vi "SVT THD and Harmonic Components (Frequency) (1 Ch).vi"(0 "complex spectrum":T9={"complex spectrum response"={"f0"=0.0, "df"=1.0, "complex spectrum"=[]}, "spectrum info"={"channel name"="", "description"="", "x-axis units"=0, "spectral info"={"spectrum type"=enum."Power [Magnitude^2]", "linear/dB"=enum."linear", "window"=0, "window size"=0, "FFT size"=0}, "engineering units"=0, "custom label"="", "dB reference [EU]"=0.0, "peak units"=enum."rms", "weighting filter"=0, "spectral density?"=FALSE, "unit label"="", "spectrum skewed?"=FALSE, "complimentary spectrum units"=enum."none"}} {"spectrum info"."x-axis units" items=["Time (s)"=0, "Frequency-CB (Hz)"=1, "Frequency-CPB (Hz)"=1248, "Frequency-Arbitrary (Hz)"=2357, "Quefrency (s)"=2, "Revolutions (rev)"=3, "Order"=4, "Speed (RPM)"=11, "Speed (rad/s)"=21, "Index"=65535]; "spectrum info"."weighting filter" items=["Linear", "A-weighting", "B-weighting", "C-weighting", "ITU-R 468-4", "Dolby", "CCITT", "C-message", "Wb", "Wc", "Wd", "We", "Wf", "Wh", "Wj", "Wk", "Wm", "AES17 20 kHz lowpass", "AES17 40 kHz lowpass", "AES17 20 kHz highpass", "AES17 40 kHz highpass"]; "spectrum info"."dB reference [EU]" format="%.2f"; "spectrum info"."engineering units" items=["custom..."=0, "V"=1, "A"=21, "C"=30, "pC"=31, "s"=32, "-"=29, "Pa"=2, "N"=20, "g"=3, "m/s^2"=4, "m/s"=5, "m"=6, "mm/s"=12, "mm"=13, "micron/s"=14, "micron"=15, "in/s^2"=7, "in/s"=8, "in"=9, "mil/s"=10, "mil"=11, "rad/s^2"=16, "rad/s"=17, "rad"=18, "deg/s^2"=26, "deg/s"=27, "deg"=28, "RPM"=22, "cycle/s^2"=23, "Hz"=24, "cycle"=25, "strain"=19]; "spectrum info"."spectral info"."window" items=["None "=0, "Hanning"=1, "Hamming"=2, "Blackman-Harris"=3, "Exact Blackman"=4, "Blackman"=5, "Flat Top"=6, "4 Term B-Harris "=7, "7 Term B-Harris"=8, "Low Sidelobe"=9, "Force - Exponential"=10, "Gaussian"=62]; "complex spectrum response"."complex spectrum" format="%.2f"; "complex spectrum response"."df" format="%.2f"; "complex spectrum response"."f0" format="%.2f"}, 2 "maximum harmonic":i32=-1, 3 "harmonics to visualize":i32[](array[numeric])=[-1], 5 "error in (no error)":errorcluster, 6 "desired units":T2, 9 "expected fundamental frequency [Hz]":dbl=-1.0 format="%.2f") -> (10 "actual maximum harmonic":i32=5, 11 "detected fundamental\nfrequency [Hz]":dbl format="%.2f", 12 "unit labels":T1, 13 "detected fundamental\namplitude":dbl format="%.2f", 14 "complex spectrum":T9={"complex spectrum response"={"f0"=0.0, "df"=1.0, "complex spectrum"=[]}, "spectrum info"={"channel name"="", "description"="", "x-axis units"=0, "spectral info"={"spectrum type"=enum."Power [Magnitude^2]", "linear/dB"=enum."linear", "window"=0, "window size"=0, "FFT size"=0}, "engineering units"=0, "custom label"="", "dB reference [EU]"=0.0, "peak units"=enum."rms", "weighting filter"=0, "spectral density?"=FALSE, "unit label"="", "spectrum skewed?"=FALSE, "complimentary spectrum units"=enum."none"}} {"spectrum info"."x-axis units" items=["Time (s)"=0, "Frequency-CB (Hz)"=1, "Frequency-CPB (Hz)"=1248, "Frequency-Arbitrary (Hz)"=2357, "Quefrency (s)"=2, "Revolutions (rev)"=3, "Order"=4, "Speed (RPM)"=11, "Speed (rad/s)"=21, "Index"=65535]; "spectrum info"."weighting filter" items=["Linear", "A-weighting", "B-weighting", "C-weighting", "ITU-R 468-4", "Dolby", "CCITT", "C-message", "Wb", "Wc", "Wd", "We", "Wf", "Wh", "Wj", "Wk", "Wm", "AES17 20 kHz lowpass", "AES17 40 kHz lowpass", "AES17 20 kHz highpass", "AES17 40 kHz highpass"]; "spectrum info"."dB reference [EU]" format="%.2f"; "spectrum info"."engineering units" items=["custom..."=0, "V"=1, "A"=21, "C"=30, "pC"=31, "s"=32, "-"=29, "Pa"=2, "N"=20, "g"=3, "m/s^2"=4, "m/s"=5, "m"=6, "mm/s"=12, "mm"=13, "micron/s"=14, "micron"=15, "in/s^2"=7, "in/s"=8, "in"=9, "mil/s"=10, "mil"=11, "rad/s^2"=16, "rad/s"=17, "rad"=18, "deg/s^2"=26, "deg/s"=27, "deg"=28, "RPM"=22, "cycle/s^2"=23, "Hz"=24, "cycle"=25, "strain"=19]; "spectrum info"."spectral info"."window" items=["None "=0, "Hanning"=1, "Hamming"=2, "Blackman-Harris"=3, "Exact Blackman"=4, "Blackman"=5, "Flat Top"=6, "4 Term B-Harris "=7, "7 Term B-Harris"=8, "Low Sidelobe"=9, "Force - Exponential"=10, "Gaussian"=62]; "complex spectrum response"."complex spectrum" format="%.2f"; "complex spectrum response"."df" format="%.2f"; "complex spectrum response"."f0" format="%.2f"}, 16 "THD":dbl format="%.2f", 17 "harmonic components":cluster{"frequency [Hz]":dbl, "amplitude":dbl}[](array[cluster]) {"amplitude" format="%.2f"; "frequency [Hz]" format="%.2f"}, 19 "error out":errorcluster)   [LabVIEW 2017, in "SoundVib_Distortion.lvlib"]
doc: "Performs a total harmonic distortion analysis, including measuring the fundamental tone and harmonics, and returns the detected fundamental frequency, detected fundamental amplitude, harmonic components, and total harmonic distortion (THD). Wire data to the <B>scaled signal [EU]</B> input to determine the polymorphic instance to use or manually select the instance.\n\nThe following formula calculates THD:\n\nTHD = H / F\n\nwhere H is the harmonic RMS level and F is the fundamental tone RMS level."
uses:
  <vilib>/addons/Sound and Vibration/svt_Distortion/SoundVib_Distortion.lvlib
  <vilib>/addons/_NISVFA/_Shared subVIs/Controls/svc_Spectrum Info.ctl
  <vilib>/addons/_NISVFA/_Shared subVIs/Controls/svc_X-Axis Units.ctl
  <vilib>/addons/_NISVFA/_Shared subVIs/Controls/svc_Spectrum Type.ctl
  <vilib>/addons/_NISVFA/_Shared subVIs/Controls/svc_Engineering Units Text Ring.ctl
  <vilib>/addons/_NISVFA/_Shared subVIs/Controls/svc_Weighting Filter Text Ring.ctl
  <vilib>/addons/_NISVFA/_Shared subVIs/Controls/svc_Complimentary Spectrum Units.ctl
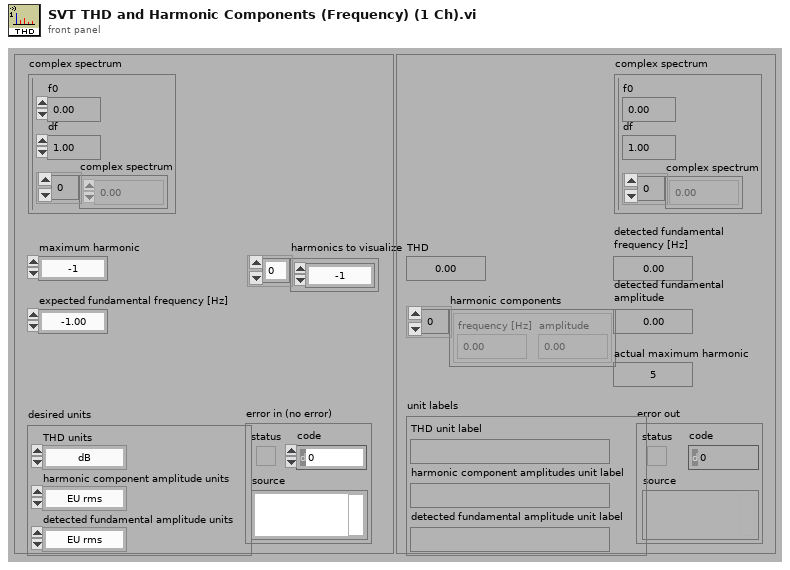
[diagram p1: front panel]
types:
  T1 = cluster{"THD unit label":string, "harmonic component amplitudes unit label":string, "detected fundamental amplitude unit label":string}
  T2 = cluster{"THD units":enum16{"dB", "linear ratio", "%"}, "harmonic component amplitude units":enum16{"EU rms", "EU peak", "EU peak-peak", "dB ref fund"}, "detected fundamental amplitude units":enum16{"EU rms", "EU peak", "EU peak-peak"}}
  T3 = typedef "svc_Spectrum Info.ctl" = cluster{"channel name":string, "description":string, "x-axis units":T4, "spectral info":cluster{"spectrum type":T5, "linear/dB":enum16{"linear", "dB"}, "window":u16, "window size":i32, "FFT size":i32}, "engineering units":T6, "custom label":string, "dB reference [EU]":dbl, "peak units":enum16{"rms", "peak", "peak-peak"}, "weighting filter":T7, "spectral density?":bool, "unit label":string, "spectrum skewed?":bool, "complimentary spectrum units":T8}
  T4 = typedef "svc_X-Axis Units.ctl" = u16
  T5 = typedef "svc_Spectrum Type.ctl" = enum16{"FFT Spectrum [complex]", "Amplitude [Magnitude]", "Power [Magnitude^2]", "Cross Spectrum [complex]", "Frequency Response [Complex]"}
  T6 = typedef "svc_Engineering Units Text Ring.ctl" = u16
  T7 = typedef "svc_Weighting Filter Text Ring.ctl" = u16
  T8 = typedef "svc_Complimentary Spectrum Units.ctl" = enum16{"none", "radians", "degrees", "cycles", "imaginary"}
  T9 = cluster{"complex spectrum response":cluster{"f0":dbl, "df":dbl, "complex spectrum":cdb[]}, "spectrum info":T3}
  T10 = cluster{"unit label":string, "unit label":string, "unit label":string}
  T11 = enum16{"EU rms", "EU peak", "EU peak-peak", "dB ref fund"}
  T12 = cluster{"SINAD [ratio]":dbl, "THD+N [ratio]":dbl, "THD":dbl}
  T13 = cluster{"detected frequency [Hz]":dbl, "detected amplitude":dbl}[]
  T14 = cluster{"frequency [Hz]":dbl, "converted harmonic amplitude":dbl}
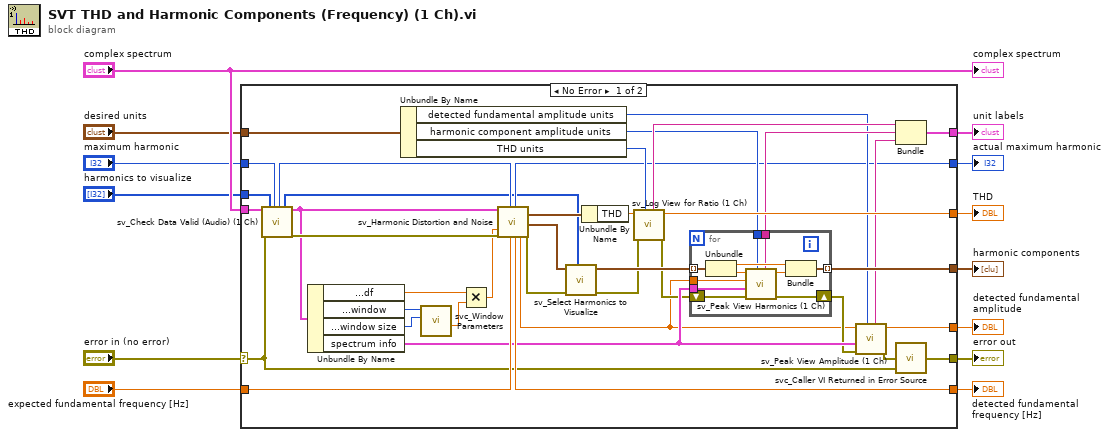
[diagram p0: block diagram]
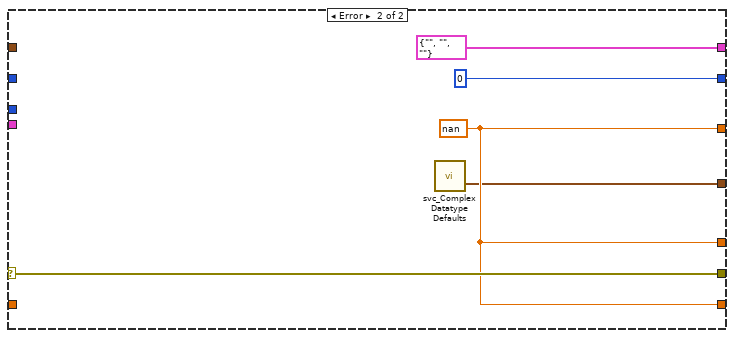
[diagram p2: hidden frame]
diagram:
  n1 = case shown="No Error" "error in (no error)" {
    selector: "error in (no error)" -> [w20 w68]
    tunnel: "complex spectrum" -> [w32 _]
    tunnel: "expected fundamental frequency [Hz]" -> [w52 _]
    tunnel: [w49 w68] -> w12
    tunnel: [w45 w67] -> w11
    tunnel: [w39 w64] -> w6
    tunnel: [w51 w67] -> w9
    tunnel: [w48 w67] -> w7
    tunnel: "maximum harmonic" -> [w33 _]
    tunnel: "harmonics to visualize" -> [w34 _]
    tunnel: "desired units" -> [w47 _]
    tunnel: [w36 T10 {"unit label"="", "unit label"="", "unit label"=""}] -> w2
    tunnel: [w35 0 ("actual maximum harmonic")] -> w1
    frame No Error {
      n2 = call <vilib>:"sv_Check Data Valid (Audio) (1 Ch).vi"("complex spectrum"=w32, "error in (no error)"=w20, "harmonics to visualize"=w34, "maximum harmonic"=w33) -> ("dup maximum harmonic"=w31:i32, "dup harmonics to visualize"=w27:i32[], "complex spectrum"=w28:T9, "error out"=w30:errorcluster)  [unwired: 8 in, 4 out]
      n3 = Unbundle By Name(w28) -> ("complex spectrum response.df"=w16:dbl, "spectrum info.spectral info.window"=w18:u16, "spectrum info.spectral info.window size"=w17:i32, "spectrum info"=w26:T3)
      n4 = Unbundle By Name(w47) -> ("detected fundamental amplitude units"=w38:enum16{"EU rms", "EU peak", "EU peak-peak"}, "harmonic component amplitude units"=w41:T11, "THD units"=w44:enum16{"dB", "linear ratio", "%"})
      n5 = call <vilib>:"svc_Window Parameters.vi"("window size"=w17, "window"=w18) -> ("6dB BW"=w15:dbl)  [unwired: 6 in, 3 out]
      n6 = Multiply(x=w16, y=w15) -> (x*y=w14:dbl)
      n7 = call <vilib>:"sv_Harmonic Distortion and Noise.vi"("complex spectrum"=w28, "advanced span [Hz]"=w14, "error in"=w30, "maximum harmonic"=w31, "approx. fund. freq. (optional)"=w52) -> ("actual maximum harmonic"=w35:i32, "detected fundamental frequency"=w51:dbl, "detected amplitude"=w21:dbl, "distortion measurements"=w46:T12, "harmonic components"=w25:T13, "error out"=w50:errorcluster)  [unwired: 7 in, 2 out]
      n8 = call <vilib>:"sv_Select Harmonics to Visualize.vi"("harmonics to visualize"=w27, "error in (no error)"=w50, "harmonic components"=w25) -> ("error out"=w22:errorcluster, "selected harmonic components"=w42:cluster{"frequency [Hz]":dbl, "amplitude":dbl}[])  [unwired: 7 in]
      n9 = Unbundle By Name(w46) -> ("THD"=w19:dbl)
      n10 = call <vilib>:"sv_Log View for Ratio (1 Ch).vi"("ratio units"=w44, "error in (no error)"=w22, "linear ratio"=w19) -> ("error out"=w23:errorcluster, "converted ratio"=w45:dbl, "unit label"=w43:string)  [unwired: 6 in]
      n11 = for {
        tunnel: w42 -> [w63] mode=indexing
        tunnel: w41 -> [w59]
        tunnel: [w58] -> w40
        tunnel: [w57] -> w39 mode=indexing
        tunnel: w26 -> [w56]
        shift-right: [w55] -> w24
        shift-left: w23 -> [w54]
        tunnel: w21 -> [w53]
        n12 = Unbundle(w63) -> ("frequency [Hz]"=w60:dbl, "amplitude"=w62:dbl)
        n13 = call <vilib>:"sv_Peak View Harmonics (1 Ch).vi"("harmonic units"=w59, "error in (no error)"=w54, "spectrum info"=w56, "fundamental amplitude [EU pk]"=w53, "harmonic amplitude [EU pk]"=w62) -> ("error out"=w55:errorcluster, "converted harmonic amplitude"=w61:dbl, "unit label"=w58:string)  [unwired: 4 in]
        n14 = Bundle("frequency [Hz]"=w60, "converted harmonic amplitude"=w61) -> (w57:T14)  [unwired: 1 in]
      }
      n15 = call <vilib>:"sv_Peak View Amplitude (1 Ch).vi"("peak units"=w38, "error in (no error)"=w24, "spectrum info"=w26, "peak amplitude [EU pk]"=w21) -> ("error out"=w29:errorcluster, "converted peak amplitude"=w48:dbl, "unit label"=w37:string)  [unwired: 5 in]
      n16 = Bundle("unit label"=w43, "unit label"=w40, "unit label"=w37) -> (w36:T10)  [unwired: 1 in]
      n17 = call <vilib>:"svc_Caller VI Returned in Error Source.vi"("warning input to caller"=w20, "error in (no error)"=w29) -> ("error out"=w49:errorcluster)  [unwired: 3 in]
    }
    frame Error {
      w67 = nan ("SINAD")
      n18 = call <vilib>:"svc_Complex Datatype Defaults.vi"() -> ("empty array of peaks"=w64:cluster{"frequency":dbl, "value":dbl}[])  [unwired: 11 in, 8 out]
    }
  }
  "error out" <- w12
  "THD" <- w11
  "detected fundamental\nfrequency [Hz]" <- w9
  "detected fundamental\namplitude" <- w7
  "harmonic components" <- w6
  "unit labels" <- w2
  "actual maximum harmonic" <- w1
  "complex spectrum" <- "complex spectrum"
